vi "createT7Inclinometer.vi"(8 "error in (no error)":errorcluster, 11 "Boot in":refnum<class "Boot.lvclass">) -> (0 "error out":errorcluster, 2 "T7Inclinometer":refnum<class "T7Inclinometer.lvclass">, 3 "Boot out":refnum<class "Boot.lvclass">)   [LabVIEW 2016, in "Boot.lvclass"]
uses:
  Boot.lvclass
  Common_RT_T7Inclinometer/T7Inclinometer/T7Inclinometer.lvclass
  Common_RT_T7Inclinometer/T7Inclinometer/T7Inclinometer.lvclass/T7Inclinometer.ctl
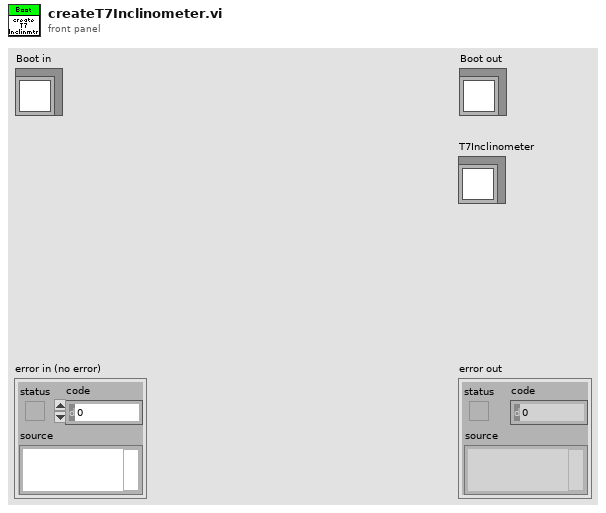
[diagram p1: front panel]
types:
  T1 = typedef "M1M3SupportSettings.lvlib/BaseT7InclinometerSettings.ctl" = cluster{"Address":u8}
  T2 = typedef "RTT7Inclinometer.lvlib/T7InclinometerData.ctl" = cluster{"Constants":T3, "Telemetry":T4, "Responses":T5, "Timestamps":T7}
  T3 = typedef "RTT7Inclinometer.lvlib/T7InclinometerConstants.ctl" = cluster{"Address":u8}
  T4 = typedef "RTT7Inclinometer.lvlib/T7InclinometerTelemetry.ctl" = cluster{"Angle":dbl}
  T5 = typedef "RTT7Inclinometer.lvlib/T7InclinometerResponses.ctl" = cluster{"ReadAngle":T6}
  T6 = typedef "RTT7Inclinometer.lvlib/T7InclinometerErrors.ctl" = enum16{"None", "InvalidFunctionCodeError", "InvalidRegisterAddressError", "InvalidCRCError", "UnknownAddressError", "UnknownFunctionError", "InvalidResponseLengthError", "UnknownError"}
  T7 = typedef "RTT7Inclinometer.lvlib/T7InclinometerTimestamps.ctl" = cluster{"ReadAngle":dbl}
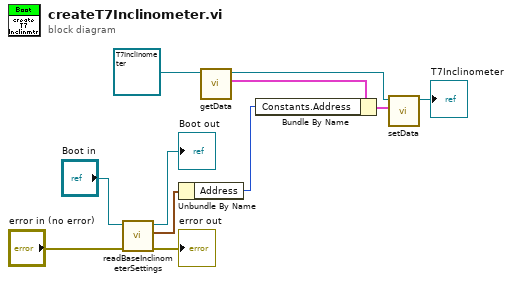
[diagram p0: block diagram]
diagram:
  n1 = call "readBaseInclinometerSettings.vi"("error in (no error)"="error in (no error)", "Boot in"="Boot in") -> ("error out"=→"error out":errorcluster, "BaseT7InclinometerSettings"=w4:T1, "Boot out"=→"Boot out":refnum<class "Boot.lvclass">)  [unwired: 7 in]
  n2 = Unbundle By Name(w4) -> ("Address"=w3:u8)
  n3 = call "getData.vi"("T7Inclinometer in"=refnum<class "T7Inclinometer.lvclass"> refnum ("RTT7Inclinometer.lvlib:T7Inclinometer.lvclass")) -> ("T7InclinometerData"=w6:T2, "T7Inclinometer out"=w7:refnum<class "T7Inclinometer.lvclass">)  [unwired: 9 in]
  n4 = Bundle By Name(cluster=w6, "Constants.Address"=w3) -> (w5:T2)
  n5 = call "setData.vi"("T7InclinometerData"=w5, "T7Inclinometer in"=w7) -> ("T7Inclinometer out"=→"T7Inclinometer":refnum<class "T7Inclinometer.lvclass">)  [unwired: 9 in]
